vi "clusters2.vi"() -> ()   [LabVIEW 2011]
panel:
  in  "Input Cluster":cluster{"Numeric":dbl, "Boolean":bool}
  in  "Boolean":bool
  in  "Numeric":dbl
  out "Output":cluster{"Numeric":dbl, "Boolean":bool}
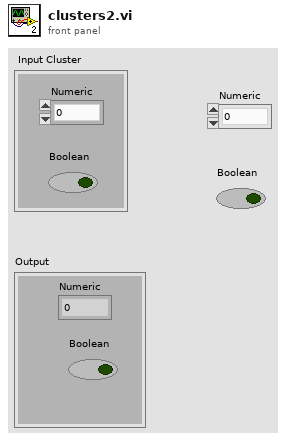
[diagram p1: front panel]
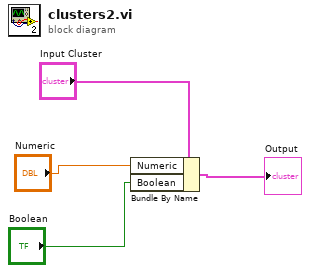
[diagram p0: block diagram]
diagram:
  n1 = Bundle By Name(cluster="Input Cluster", "Numeric"="Numeric", "Boolean"="Boolean") -> (→"Output":cluster{"Numeric":dbl, "Boolean":bool})
